vi "Copy lvlib To Disk.vi"(8 "Library Folder Path":path, 9 "Template Library Path":path, 10 "Application Instance":refnum<vi>) -> (0 "error out":errorcluster)   [LabVIEW 2021, in "_Template.lvlib" / "Script.lvlib"]
uses:
  Script.lvlib
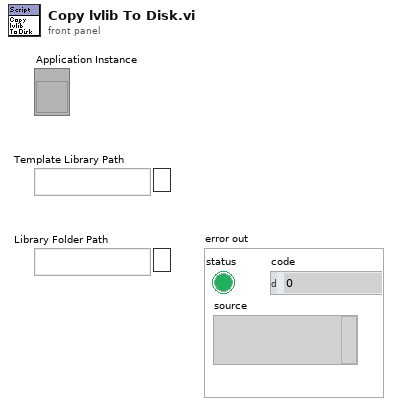
[diagram p1: front panel]
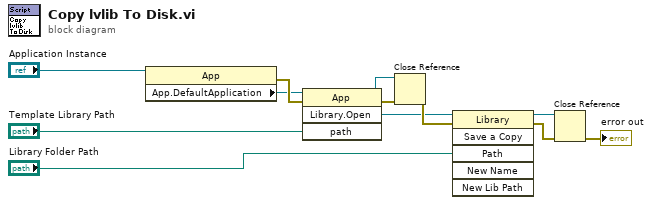
[diagram p0: block diagram]
diagram:
  n1 = property class="App"(reference="Application Instance") -> (error out=w11:errorcluster, "App.DefaultApplication"=w7:refnum<vi>)  [unwired: 1 in, 1 out]
  n2 = invoke class="App" method="Library.Open"(reference=w7, error in=w11, "path"="Template Library Path") -> (reference out=w6:refnum<vi>, error out=w12:errorcluster, "Open Library"=w9:refnum<vi>)  [unwired: 1 in, 1 out]
  n3 = Close Reference(reference=w6, error in (no error)=w12) -> (error out=w10:errorcluster)
  n4 = invoke class="Library" method="Save a Copy"(reference=w9, error in=w10, "Path"="Library Folder Path") -> (reference out=w8:refnum<vi>, error out=w5:errorcluster)  [unwired: 3 in, 4 out]
  n5 = Close Reference(reference=w8, error in (no error)=w5) -> (error out=→"error out":errorcluster)
